vi "MU Get DLL Version.vi"(8 "error in (no error)":errorcluster) -> (0 "error out (no error)":errorcluster, 2 "version":u32[](array[numeric]), 3 "function return":u32)   [LabVIEW 2017, in "MU_3SL_interface.lvlib"]
uses:
  MU_3SL_interface.lvlib
  lib/MU_3SL_interface.dll
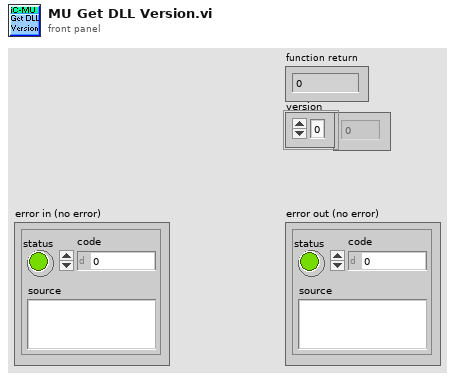
[diagram p1: front panel]
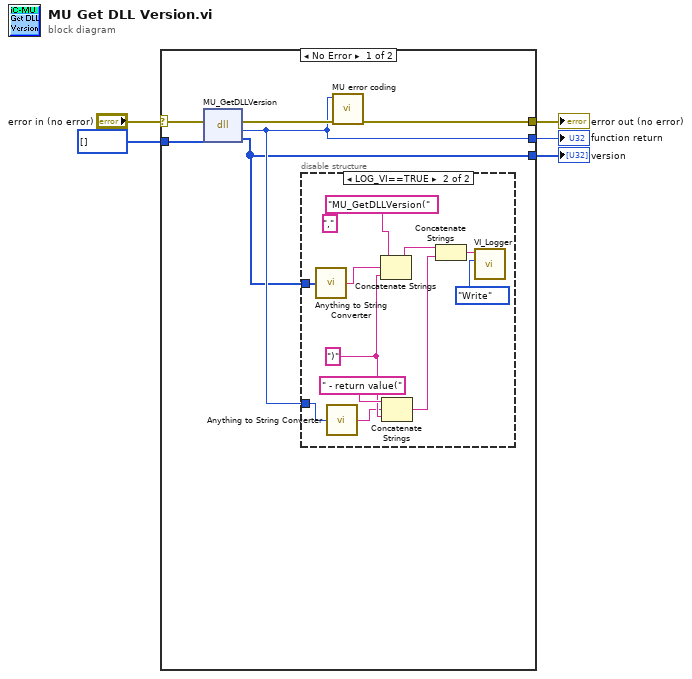
[diagram p0: block diagram]
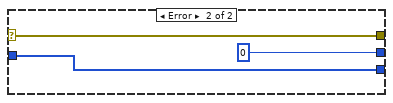
[diagram p3: hidden frame]
diagram:
  n1 = case shown="No Error" "error in (no error)" {
    selector: "error in (no error)" -> [w9 w25]
    tunnel: [w7 u32 0 ("return type")] -> w5
    tunnel: [w6 w23] -> w1
    tunnel: [w10 w25] -> w4
    tunnel: u32[] [] ("pulDllVersion") -> [w8 w23]
    frame No Error {
      n2 = dll-call lib="C:/Users/bes/AppData/Roaming/work/mu_9so/icsubmodules/soft_mu_3sl_master/lv_interface/lib/MU_3SL_interface**.*" fn="MU_GetDLLVersion"(error in=w9, "version"=w8) -> (error out=w11:errorcluster, "return type"=w7:u32, "version"=w6:u32[])  [unwired: 2 in, 1 out]
      n3 = disable-structure shown="LOG_VI==TRUE" {
        disable-tunnel: w7 -> [_ w13]
        disable-tunnel: w6 -> [_ w15]
        frame condition #0 {
        }
        frame condition #1 (active) {
          w16 = ")" ("string")
          (unwired) "," ("string")
          n4 = call "Anything to String Converter.vi"("anything"=w15) -> ("String"=w14:string)
          n5 = call "Anything to String Converter.vi"("anything"=w13) -> ("String"=w12:string)
          n6 = Concatenate Strings("MU_GetDLLVersion(" ("Info in"), w14, w16) -> (w20:string)
          n7 = Concatenate Strings(" - return value(" ("string"), w12, w16) -> (w19:string)
          n8 = Concatenate Strings(w20, w19) -> (w18:string)
          n9 = call "VI_Logger.vi"("Action (Read)"=enum16{"Write", "Read"}."Write", "Info in"=w18) -> ()  [unwired: 8 in, 2 out]
        }
      }
      n10 = call "MU error coding.vi"("error in (no error)"=w11, "function return in"=w7) -> ("error out"=w10:errorcluster)  [unwired: 9 in]
    }
    frame Error {
    }
  }
  "function return" <- w5
  "version" <- w1
  "error out (no error)" <- w4
